vi "MAG_DATA_READ.vi"() -> ()   [LabVIEW 2011]
uses:
  <vilib>/Native 3D Graph/xcontrol/3DPC_SurfacePlot.xctl
  <vilib>/Utility/file.llb/Write To Spreadsheet File (DBL).vi
  <vilib>/Analysis/coordinate.llb/3D Coordinate Conversion (Scalar).vi
  <vilib>/Analysis/NI_AALPro.lvlib
  <vilib>/Analysis/NI_AALBase.lvlib
  <vilib>/Utility/miscctls.llb/LVRangeTypeDef.ctl
panel:
  in  "Tab Control":T1(tab)
  in  "VISA-Ressourcenname":refnum<visa-resource-name>="COM7"
  in  "iIndex":u32
  in  "y":dbl=-0.158
  in  "z":dbl=0.065
  in  "x":dbl=0.115
  out "DeviceID":u8 format="%02x"
  out "X_Y_Range":dbl
  out "Z_Range":dbl
  out "Magnitude":dbl[][](graph)
  out "3D Graph":refnum<class "Base Datatype.lvclass">[](xcontrol)
  out "Theta":dbl[][](graph)
  out "Phi":dbl[][](graph)
  out "Temp":dbl[][](graph)
  in  "phi_step":dbl=5.0
  in  "phi_end":dbl=90.0
  in  "phi_start":dbl=-90.0
  in  "theta_step":dbl=5.0
  in  "theta_end":dbl=360.0
  in  "theta_start":dbl
  out "phi":dbl
  out "theta":dbl
  in  "Magnitude (mT)":dbl
  in  "stop":bool
  out "data":T2 {"Temperature 2" format="%.1f"; "Z" format="%0.2f"; "Y" format="%0.2f"; "X" format="%0.2f"; "Magnitude (mT)" format="%#.4f"}
  # "Offsets"
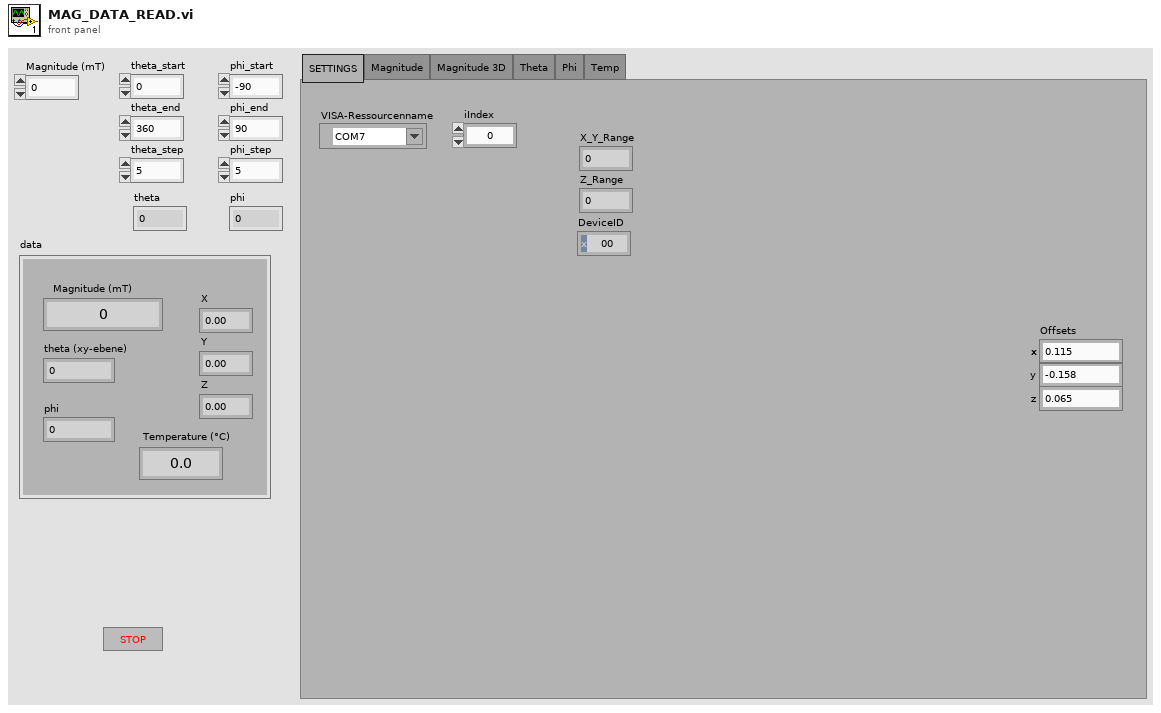
[diagram p1: front panel]
types:
  T1 = enum32{"SETTINGS", "Magnitude", "Magnitude 3D", "Theta", "Phi", "Temp"}
  T2 = cluster{"X":dbl, "Y":dbl, "Z":dbl, "Magnitude (mT)":dbl, "theta (xy-ebene)":dbl, "phi":dbl, "Temperature 2":dbl}
  T3 = typedef "LVRangeTypeDef.ctl" = cluster{"Minimum":dbl, "Maximum":dbl, "Increment":dbl, "Minor Increment":dbl, "Start":dbl}
  T4 = enum8{"Standard I2C 3-byte read command", "1-byte I2C read command for 16bit sensor data and conversion\nstatus", "1-byte I2C read command for 8 bit sensor MSB data and\nconversion status", "Reserved"}
  T5 = cluster{"Temperature (°C)":dbl, "x (mT)":dbl, "y (mT)":dbl, "z (mT)":dbl}
  T6 = cluster{"I2C_RD":enum8{"Standard I2C 3-byte read command", "1-byte I2C read command for 16bit sensor data and conversion\nstatus", "1-byte I2C read command for 8 bit sensor MSB data and\nconversion status", "Reserved"}, "CONV_AVG":enum8{"1x average, 10.0-kSPS (3-axes) or 20-kSPS (1 axis)", "2x average, 5.7-kSPS (3-axes) or 13.3-kSPS (1 axis)", "4x average, 3.1-kSPS (3-axes) or 8.0-kSPS (1 axis)", "8x average, 1.6-kSPS (3-axes) or 4.4-kSPS (1 axis)", "16x average, 0.8-kSPS (3-axes) or 2.4-kSPS (1 axis)", "32x average, 0.4-kSPS (3-axes) or 1.2-kSPS (1 axis)"}, "MAG_TEMPCO":enum8{"0 %/°C (No temperature compensation)", "0.12 %/°C (NdBFe)", "0.03 %/°C (SmCo)", "0.20 %/°C (Ceramic)"}, "CRC_EN":enum8{"CRC disabled", "CRC enabled"}}
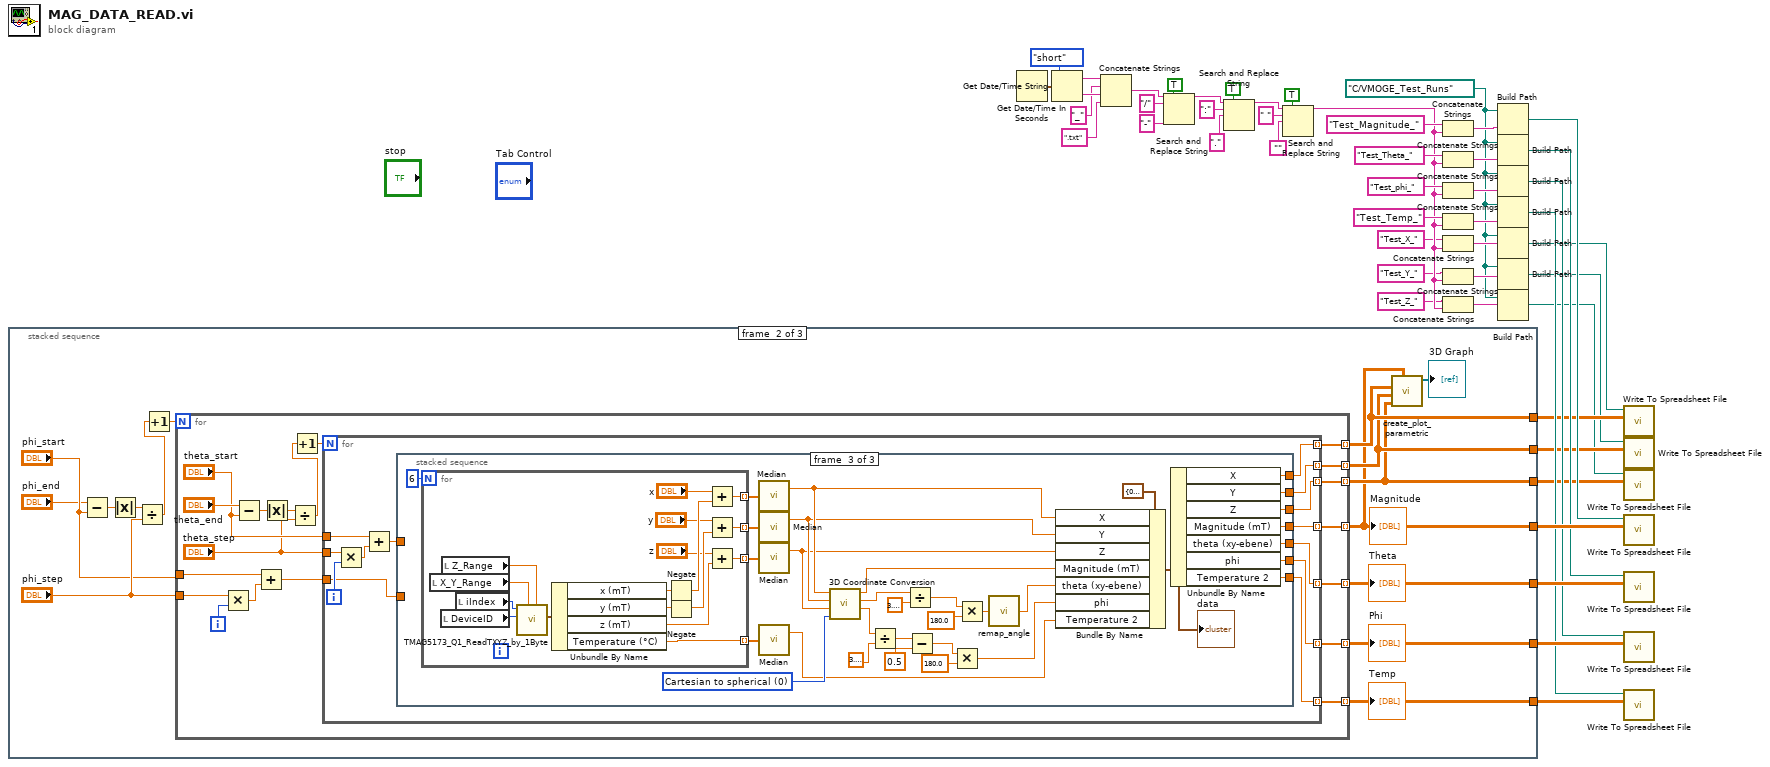
[diagram p0: block diagram]
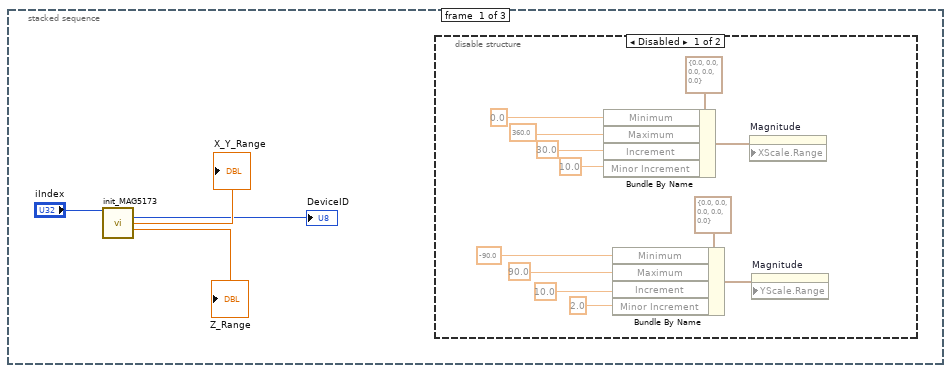
[diagram p2: hidden frame]
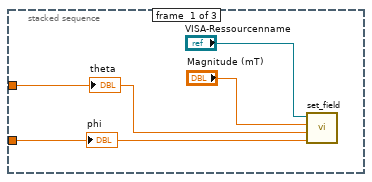
[diagram p4: hidden frame]
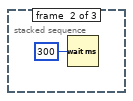
[diagram p5: hidden frame]
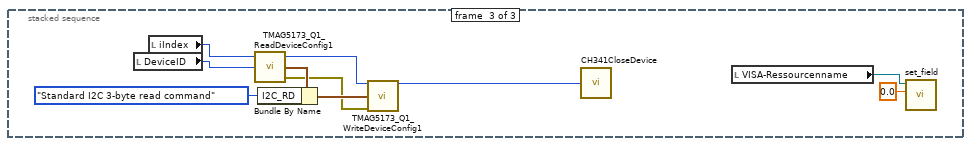
[diagram p6: hidden frame]
diagram:
  w1 = path "C:/VMOGE_Test_Runs" ("file path (dialog if empty)")
  n1 = stacked-sequence {
    tunnel: [_ w65 _] -> w48
    tunnel: [_ w71 _] -> w22
    tunnel: [_ w72 _] -> w21
    tunnel: [_ w70 _] -> w20
    tunnel: [_ w68 _] -> w12
    tunnel: [_ w67 _] -> w13
    tunnel: [_ w66 _] -> w14
    frame #0 {
      n2 = call "init_MAG5173.vi"("iIndex"="iIndex") -> ("DeviceID"=→"DeviceID":u8, "X_Y_Range"=→"X_Y_Range":dbl, "Z_Range"=→"Z_Range":dbl)  [unwired: 10 in, 2 out]
      n3 = disable-structure shown="Disabled" {
        frame Disabled {
          n4 = Bundle By Name(cluster=T3 {"Minimum"=0.0, "Maximum"=0.0, "Increment"=0.0, "Minor Increment"=0.0, "Start"=0.0} ("X Scale.Range"), "Minimum"=0.0, "Maximum"=360.0 ("Minimum"), "Increment"=30.0 ("Minimum"), "Minor Increment"=10.0) -> (w63:T3)
          n5 = Bundle By Name(cluster=T3 {"Minimum"=0.0, "Maximum"=0.0, "Increment"=0.0, "Minor Increment"=0.0, "Start"=0.0} ("X Scale.Range"), "Minimum"=-90.0, "Maximum"=90.0 ("Minimum"), "Increment"=10.0 ("Minimum"), "Minor Increment"=2.0) -> (w61:T3)
          n6 = property on="Magnitude" class="IntGraph (strict)"("XScale.Range"=w63) -> ()  [unwired: 2 in, 2 out]
          n7 = property on="Magnitude" class="IntGraph (strict)"("YScale.Range"=w61) -> ()  [unwired: 2 in, 2 out]
        }
        frame Enabled {
        }
      }
    }
    frame #1 {
      n8 = Subtract(x="phi_end", y="phi_start") -> (x-y=w75:dbl)
      n9 = Absolute Value(x=w75) -> (abs(x)=w73:dbl)
      n10 = Divide(x=w73, y="phi_step") -> (x/y=w76:dbl)
      n11 = Increment(x=w76) -> (x+1=w77:dbl)
      n12 = for {
        N: w77 -> [_]
        tunnel: "phi_start" -> [w96]
        tunnel: "phi_step" -> [w97]
        tunnel: [w93] -> w65 mode=indexing
        tunnel: [w85] -> w71 mode=indexing
        tunnel: [w84] -> w70 mode=indexing
        tunnel: [w83] -> w72 mode=indexing
        tunnel: [w82] -> w68 mode=indexing
        tunnel: [w81] -> w67 mode=indexing
        tunnel: [w80] -> w66 mode=indexing
        i -> [w98]
        n13 = Multiply(x=w97, y=w98) -> (x*y=w95:dbl)
        n14 = Subtract(x="theta_end", y="theta_start") -> (x-y=w91:dbl)
        n15 = Add(x=w96, y=w95) -> (x+y=w94:dbl)
        n16 = Absolute Value(x=w91) -> (abs(x)=w90:dbl)
        n17 = Divide(x=w90, y="theta_step") -> (x/y=w89:dbl)
        n18 = Increment(x=w89) -> (x+1=w86:dbl)
        n19 = for {
          N: w86 -> [_]
          tunnel: w94 -> [w102]
          tunnel: [w107] -> w93 mode=indexing
          tunnel: "theta_start" -> [w108]
          tunnel: "theta_step" -> [w111]
          tunnel: [w106] -> w85 mode=indexing
          tunnel: [w104] -> w84 mode=indexing
          tunnel: [w105] -> w83 mode=indexing
          tunnel: [w101] -> w82 mode=indexing
          tunnel: [w100] -> w81 mode=indexing
          tunnel: [w99] -> w80 mode=indexing
          i -> [w110]
          n20 = Multiply(x=w111, y=w110) -> (x*y=w109:dbl)
          n21 = Add(x=w108, y=w109) -> (x+y=w103:dbl)
          n22 = stacked-sequence {
            tunnel: w102 -> [w113 _ _]
            tunnel: w103 -> [w112 _ _]
            tunnel: [_ _ w139] -> w107
            tunnel: [_ _ w137] -> w106
            tunnel: [_ _ w136] -> w104
            tunnel: [_ _ w135] -> w105
            tunnel: [_ _ w120] -> w101
            tunnel: [_ _ w119] -> w100
            tunnel: [_ _ w118] -> w99
            frame #0 {
              n23 = call "set_field.vi"("phi"=w113, "theta (xy-ebene)"=w112, "Magnitude (mT)"="Magnitude (mT)", "VISA-Ressourcenname"="VISA-Ressourcenname") -> ()  [unwired: 8 in]
              "theta" <- w112
              "phi" <- w113
            }
            frame #1 {
              n24 = Wait (ms)(milliseconds to wait=u32 300) -> ()  [unwired: 1 out]
            }
            frame #2 {
              w149 = u16 0 items=["Cartesian to spherical", "spherical to Cartesian", "Cartesian to cylindrical", "cylindrical to Cartesian", "spherical to cylindrical", "cylindrical to spherical"] ("conversion type")
              n25 = for {
                N: 6 -> [_]
                tunnel: [w158] -> w146 mode=indexing
                tunnel: [w157] -> w147 mode=indexing
                tunnel: [w156] -> w148 mode=indexing
                tunnel: [w155] -> w145 mode=indexing
                n26 = local read "X_Y_Range"() -> (w151:dbl)
                n27 = local read "DeviceID"() -> (w165:u8)
                n28 = local read "Z_Range"() -> (w150:dbl)
                n29 = local read "iIndex"() -> (w166:u32)
                n30 = call <userlib>:"TMAG5173_Q1_ReadTXYZ_by_1Byte.vi"("z-Range"=w150, "xy-Range"=w151, "DeviceID"=w165, "iIndex"=w166) -> ("Data"=w164:T5)  [unwired: 4 in, 3 out]
                n31 = Unbundle By Name(w164) -> ("x (mT)"=w163:dbl, "y (mT)"=w162:dbl, "z (mT)"=w159:dbl, "Temperature (°C)"=w155:dbl)
                n32 = Negate(x=w163) -> (-x=w160:dbl)
                n33 = Negate(x=w162) -> (-x=w161:dbl)
                n34 = Add(x="x", y=w160) -> (x+y=w158:dbl)
                n35 = Add(x="y", y=w161) -> (x+y=w157:dbl)
                n36 = Add(x="z", y=w159) -> (x+y=w156:dbl)
              }
              n37 = call <vilib>:"Median.vi"("X"=w146) -> ("median"=w144:dbl)  [unwired: 1 out]
              n38 = call <vilib>:"Median.vi"("X"=w147) -> ("median"=w143:dbl)  [unwired: 1 out]
              n39 = call <vilib>:"Median.vi"("X"=w148) -> ("median"=w142:dbl)  [unwired: 1 out]
              n40 = call <vilib>:"Median.vi"("X"=w145) -> ("median"=w134:dbl)  [unwired: 1 out]
              n41 = call-poly <vilib>:"3D Coordinate Conversion.vi"("conversion type"=w149, "axis 3"=w142, "axis 2"=w143, "axis 1"=w144) -> ("axis 3 out"=w127:dbl, "axis 2 out"=w126:dbl, "axis 1 out"=w141:dbl)  [unwired: 4 in, 1 out]
              n42 = Divide(x=w127, y=3.141592653589793) -> (x/y=w129:dbl)
              n43 = Divide(x=w126, y=3.141592653589793) -> (x/y=w123:dbl)
              n44 = Subtract(x=w129, y=0.5) -> (x-y=w128:dbl)
              n45 = Multiply(x=w128, y=180.0) -> (x*y=w124:dbl)
              n46 = Multiply(x=w123, y=180.0) -> (x*y=w122:dbl)
              n47 = call "remap_angle.vi"("in (-180..+180)"=w122) -> ("out (0.360)"=w121:dbl)
              n48 = Bundle By Name(cluster=T2 {"X"=0.0, "Y"=0.0, "Z"=0.0, "Magnitude (mT)"=0.0, "theta (xy-ebene)"=0.0, "phi"=0.0, "Temperature 2"=0.0} ("data"), "X"=w144, "Y"=w143, "Z"=w142, "Magnitude (mT)"=w141, "theta (xy-ebene)"=w121, "phi"=w124, "Temperature 2"=w134) -> (w138:T2)
              "data" <- w138
              n49 = Unbundle By Name(w138) -> ("X"=w120:dbl, "Y"=w119:dbl, "Z"=w118:dbl, "Magnitude (mT)"=w139:dbl, "theta (xy-ebene)"=w137:dbl, "phi"=w136:dbl, "Temperature 2"=w135:dbl)
            }
          }
        }
      }
      "Magnitude" <- w65
      "Theta" <- w71
      "Phi" <- w70
      "Temp" <- w72
      n50 = call <vilib>:"create_plot_parametric.vi"("color matrix"=w65, "z matrix"=w66, "y matrix"=w67, "x matrix"=w68) -> ("plots out"=→"3D Graph":refnum<class "Base Datatype.lvclass">[])  [unwired: 2 in, 5 out]
    }
    frame #2 {
      n51 = local read "DeviceID"() -> (w170:u8)
      n52 = local read "iIndex"() -> (w171:u32)
      n53 = call <userlib>:"TMAG5173_Q1_ReadDeviceConfig1.vi"("DeviceID"=w170, "iIndex"=w171) -> ("error out"=w172:errorcluster, "Device_Config_1"=w176:T6, "oIndex"=w173:u32)  [unwired: 1 in]
      n54 = Bundle By Name(cluster=w176, "I2C_RD"=T4."Standard I2C 3-byte read command") -> (w175:T6)
      n55 = call <userlib>:"TMAG5173_Q1_WriteDeviceConfig1.vi"("iIndex"=w173, "Device_Config_1"=w175, "error in (no error)"=w172) -> ("oIndex"=w169:u32)  [unwired: 10 in, 2 out]
      n56 = call <userlib>:"CH341CloseDevice.vi"("iIndex"=w169) -> ()  [unwired: 1 in]
      n57 = local read "VISA-Ressourcenname"() -> (w167:refnum<visa-resource-name>)
      n58 = call "set_field.vi"("Magnitude (mT)"=0.0, "VISA-Ressourcenname"=w167) -> ()  [unwired: 10 in]
    }
  }
  n59 = Get Date/Time In Seconds() -> (seconds since 1Jan1904=w47:timestamp)
  n60 = Get Date/Time String(date format (0)=enum16{"short", "long", "abbreviated"}."short", seconds (now)=w47) -> (date string=w45:string, time string=w41:string)  [unwired: 1 in]
  n61 = Concatenate Strings(w45, "_" ("string"), w41, ".txt" ("string")) -> (w44:string)
  n62 = Search and Replace String(replace all?=TRUE ("replace all? (F)"), input string=w44, search string="/", replace string="-" ("replace string (\"\")")) -> (result string=w38:string)  [unwired: 4 in, 3 out]
  n63 = Search and Replace String(replace all?=TRUE ("replace all? (F)"), input string=w38, search string=":", replace string="." ("replace string (\"\")")) -> (result string=w34:string)  [unwired: 4 in, 3 out]
  n64 = Search and Replace String(replace all?=TRUE ("replace all? (F)"), input string=w34, search string=" ", replace string="") -> (result string=w11:string)  [unwired: 4 in, 3 out]
  n65 = Concatenate Strings("Test_Magnitude_" ("name or relative path"), w11) -> (w30:string)
  n66 = Concatenate Strings("Test_Theta_" ("name or relative path"), w11) -> (w27:string)
  n67 = Concatenate Strings("Test_phi_" ("name or relative path"), w11) -> (w26:string)
  n68 = Concatenate Strings("Test_Temp_" ("name or relative path"), w11) -> (w23:string)
  n69 = Concatenate Strings("Test_X_" ("name or relative path"), w11) -> (w5:string)
  n70 = Concatenate Strings("Test_Y_" ("name or relative path"), w11) -> (w6:string)
  n71 = Concatenate Strings("Test_Z_" ("name or relative path"), w11) -> (w7:string)
  n72 = Build Path(base path=w1, name or relative path=w30) -> (appended path=w31:path)
  n73 = Build Path(base path=w1, name or relative path=w27) -> (appended path=w19:path)
  n74 = Build Path(base path=w1, name or relative path=w26) -> (appended path=w18:path)
  n75 = Build Path(base path=w1, name or relative path=w23) -> (appended path=w17:path)
  n76 = Build Path(base path=w1, name or relative path=w5) -> (appended path=w2:path)
  n77 = Build Path(base path=w1, name or relative path=w6) -> (appended path=w3:path)
  n78 = Build Path(base path=w1, name or relative path=w7) -> (appended path=w4:path)
  n79 = call-poly <vilib>:"Write To Spreadsheet File.vi"("2D data"=w12, "file path (dialog if empty)"=w2) -> ()  [unwired: 6 in, 1 out]
  n80 = call-poly <vilib>:"Write To Spreadsheet File.vi"("2D data"=w13, "file path (dialog if empty)"=w3) -> ()  [unwired: 6 in, 1 out]
  n81 = call-poly <vilib>:"Write To Spreadsheet File.vi"("2D data"=w14, "file path (dialog if empty)"=w4) -> ()  [unwired: 6 in, 1 out]
  n82 = call-poly <vilib>:"Write To Spreadsheet File.vi"("2D data"=w48, "file path (dialog if empty)"=w31) -> ()  [unwired: 6 in, 1 out]
  n83 = call-poly <vilib>:"Write To Spreadsheet File.vi"("2D data"=w22, "file path (dialog if empty)"=w19) -> ()  [unwired: 6 in, 1 out]
  n84 = call-poly <vilib>:"Write To Spreadsheet File.vi"("2D data"=w20, "file path (dialog if empty)"=w18) -> ()  [unwired: 6 in, 1 out]
  n85 = call-poly <vilib>:"Write To Spreadsheet File.vi"("2D data"=w21, "file path (dialog if empty)"=w17) -> ()  [unwired: 6 in, 1 out]
